vi "Init Module.vi"(8 "error in (no error) 4":errorcluster, 10 "UI COnfiguration  3":T2, 11 "DB Reference In":T4) -> (0 "error out":errorcluster)   [LabVIEW 2015, in "Copy of Untitled Library 1.lvlib"]
uses:
  Copy of Untitled Library 1.lvlib
  <vilib>/addons/database/Connection.llb/Conn ObjectReference.ctl
  <userlib>/origin_lib_main/userlogin_lib/Control/Queue and Caller MSG.ctl
  Controls/FGV Cluster Data.ctl
  Controls/Enum Constant.ctl
  <userlib>/origin_lib_main/ui_msg_lib/CTRL/Display MSG Types.ctl
  <vilib>/addons/database/Connection.llb/DB Tools Open Connec (String).vi
  <vilib>/addons/database/NI_Database_API.lvlib
  <userlib>/origin_lib_main/db_interface/DB Interface.lvlib
  <userlib>/origin_lib_main/ui_msg_lib/MSG Library.lvlib
panel:
  in  "Data In":T3
  in  "UI COnfiguration  2":T5
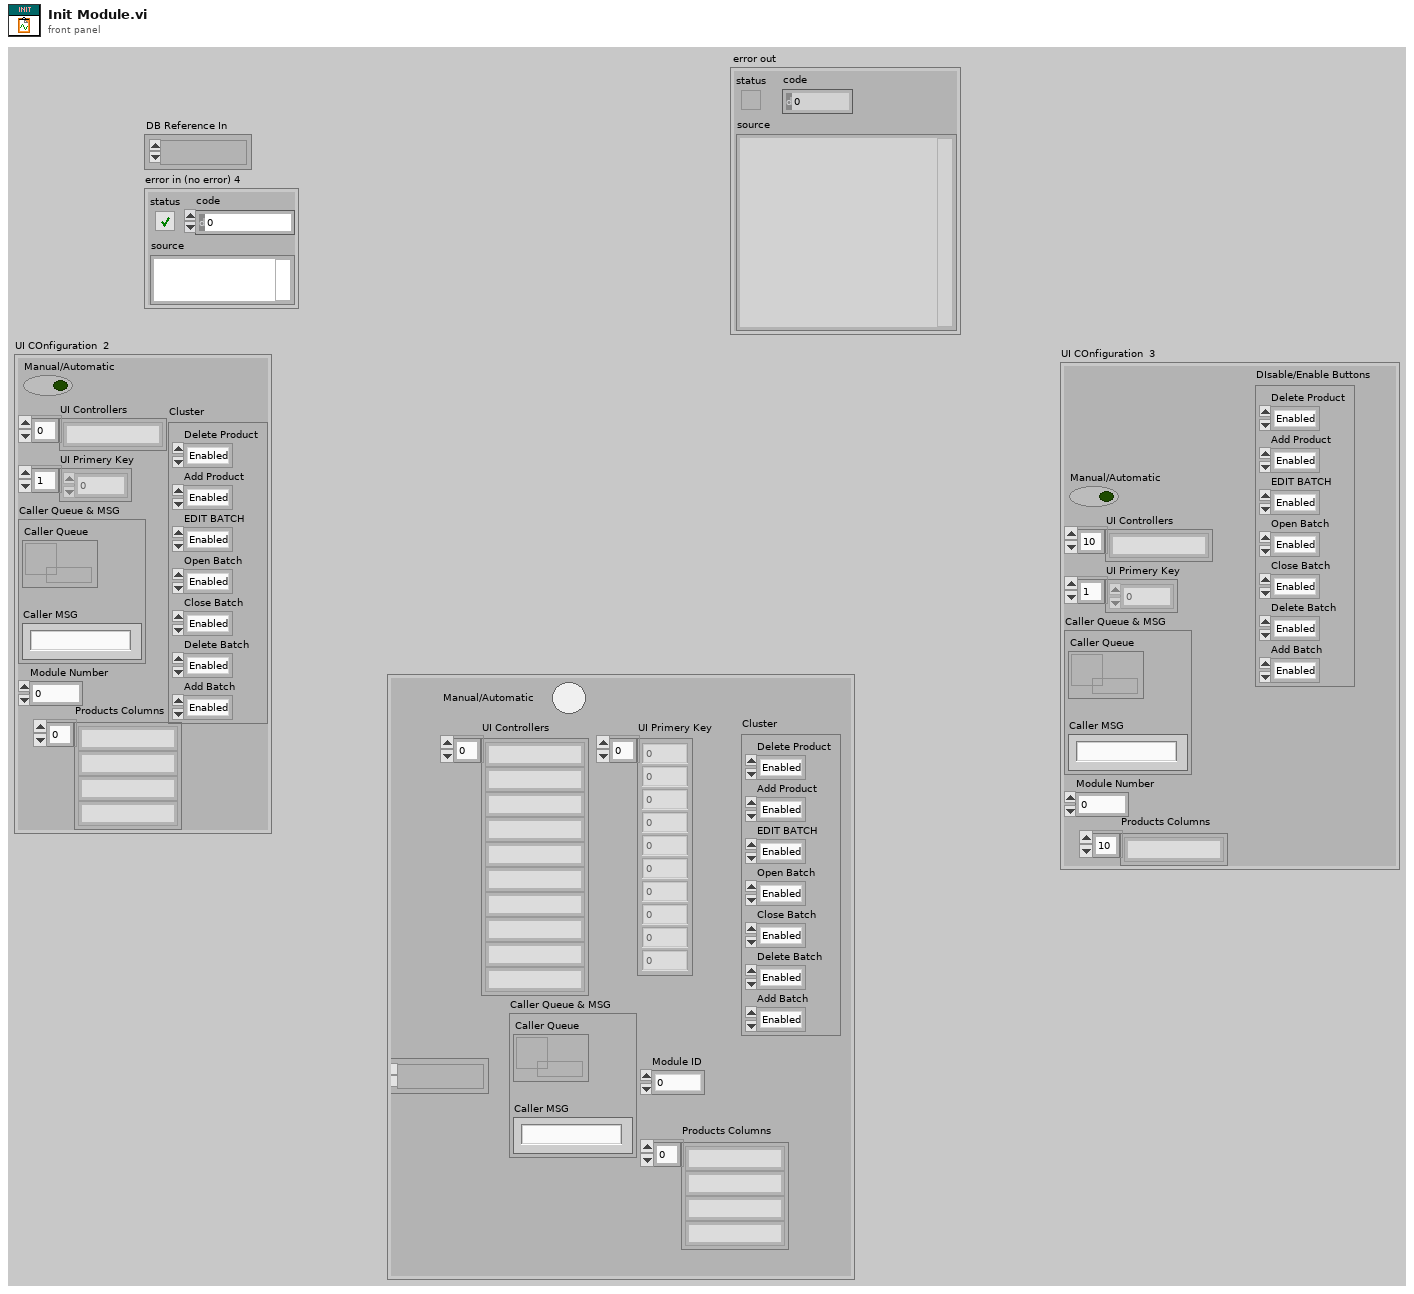
[diagram p1: front panel]
types:
  T1 = typedef "Queue and Caller MSG.ctl" = cluster{"Caller Queue":refnum<queue>, "Caller MSG":string}
  T2 = cluster{"Manual/Automatic":bool, "UI Controllers ":string[], "UI Primery Key ":dbl[], "Caller Queue & MSG":T1, "Module Number":dbl, "Products Columns":string[], "DIsable/Enable Buttons":cluster{"Delete Product":enum8{"Enabled", "Disabled", "Disabled and Grayed Out"}, "Add Product ":enum8{"Enabled", "Disabled", "Disabled and Grayed Out"}, "EDIT BATCH":enum8{"Enabled", "Disabled", "Disabled and Grayed Out"}, "Open Batch ":enum8{"Enabled", "Disabled", "Disabled and Grayed Out"}, "Close Batch":enum8{"Enabled", "Disabled", "Disabled and Grayed Out"}, "Delete Batch":enum8{"Enabled", "Disabled", "Disabled and Grayed Out"}, "Add Batch ":enum8{"Enabled", "Disabled", "Disabled and Grayed Out"}}}
  T3 = typedef "FGV Cluster Data.ctl" = cluster{"Manual/Automatic":bool, "UI Controllers ":string[], "UI Primery Key ":dbl[], "Caller Queue & MSG":T1, "Module ID":dbl, "DB Reference In":T4, "Products Columns":string[], "Cluster":cluster{"Delete Product":enum8{"Enabled", "Disabled", "Disabled and Grayed Out"}, "Add Product ":enum8{"Enabled", "Disabled", "Disabled and Grayed Out"}, "EDIT BATCH":enum8{"Enabled", "Disabled", "Disabled and Grayed Out"}, "Open Batch ":enum8{"Enabled", "Disabled", "Disabled and Grayed Out"}, "Close Batch":enum8{"Enabled", "Disabled", "Disabled and Grayed Out"}, "Delete Batch":enum8{"Enabled", "Disabled", "Disabled and Grayed Out"}, "Add Batch ":enum8{"Enabled", "Disabled", "Disabled and Grayed Out"}}}
  T4 = typedef "NI_Database_API.lvlib/Conn ObjectReference.ctl" = refnum<k1>
  T5 = cluster{"Manual/Automatic":bool, "UI Controllers ":string[], "UI Primery Key ":dbl[], "Caller Queue & MSG":T1, "Module Number":dbl, "Products Columns":string[], "Cluster":cluster{"Delete Product":enum8{"Enabled", "Disabled", "Disabled and Grayed Out"}, "Add Product ":enum8{"Enabled", "Disabled", "Disabled and Grayed Out"}, "EDIT BATCH":enum8{"Enabled", "Disabled", "Disabled and Grayed Out"}, "Open Batch ":enum8{"Enabled", "Disabled", "Disabled and Grayed Out"}, "Close Batch":enum8{"Enabled", "Disabled", "Disabled and Grayed Out"}, "Delete Batch":enum8{"Enabled", "Disabled", "Disabled and Grayed Out"}, "Add Batch ":enum8{"Enabled", "Disabled", "Disabled and Grayed Out"}}}
  T6 = enum32{"Bad", "Idle", "Run top level", "Running"}
  T7 = typedef "Enum Constant.ctl" = enum16{"Init", "Read", "Write"}
  T8 = typedef "MSG Library.lvlib/Display MSG Types.ctl" = enum16{"Display MSG 1", "Display MSG 2", "Display MSG Load", "End MSG Load ", "Display 2 STR MSG"}
  T9 = cluster{"Delete Product":enum8{"Enabled", "Disabled", "Disabled and Grayed Out"}, "Add Product ":enum8{"Enabled", "Disabled", "Disabled and Grayed Out"}, "EDIT BATCH":enum8{"Enabled", "Disabled", "Disabled and Grayed Out"}, "Open Batch ":enum8{"Enabled", "Disabled", "Disabled and Grayed Out"}, "Close Batch":enum8{"Enabled", "Disabled", "Disabled and Grayed Out"}, "Delete Batch":enum8{"Enabled", "Disabled", "Disabled and Grayed Out"}, "Add Batch ":enum8{"Enabled", "Disabled", "Disabled and Grayed Out"}}
  T10 = typedef "FGV Data.ctl" = T3[]
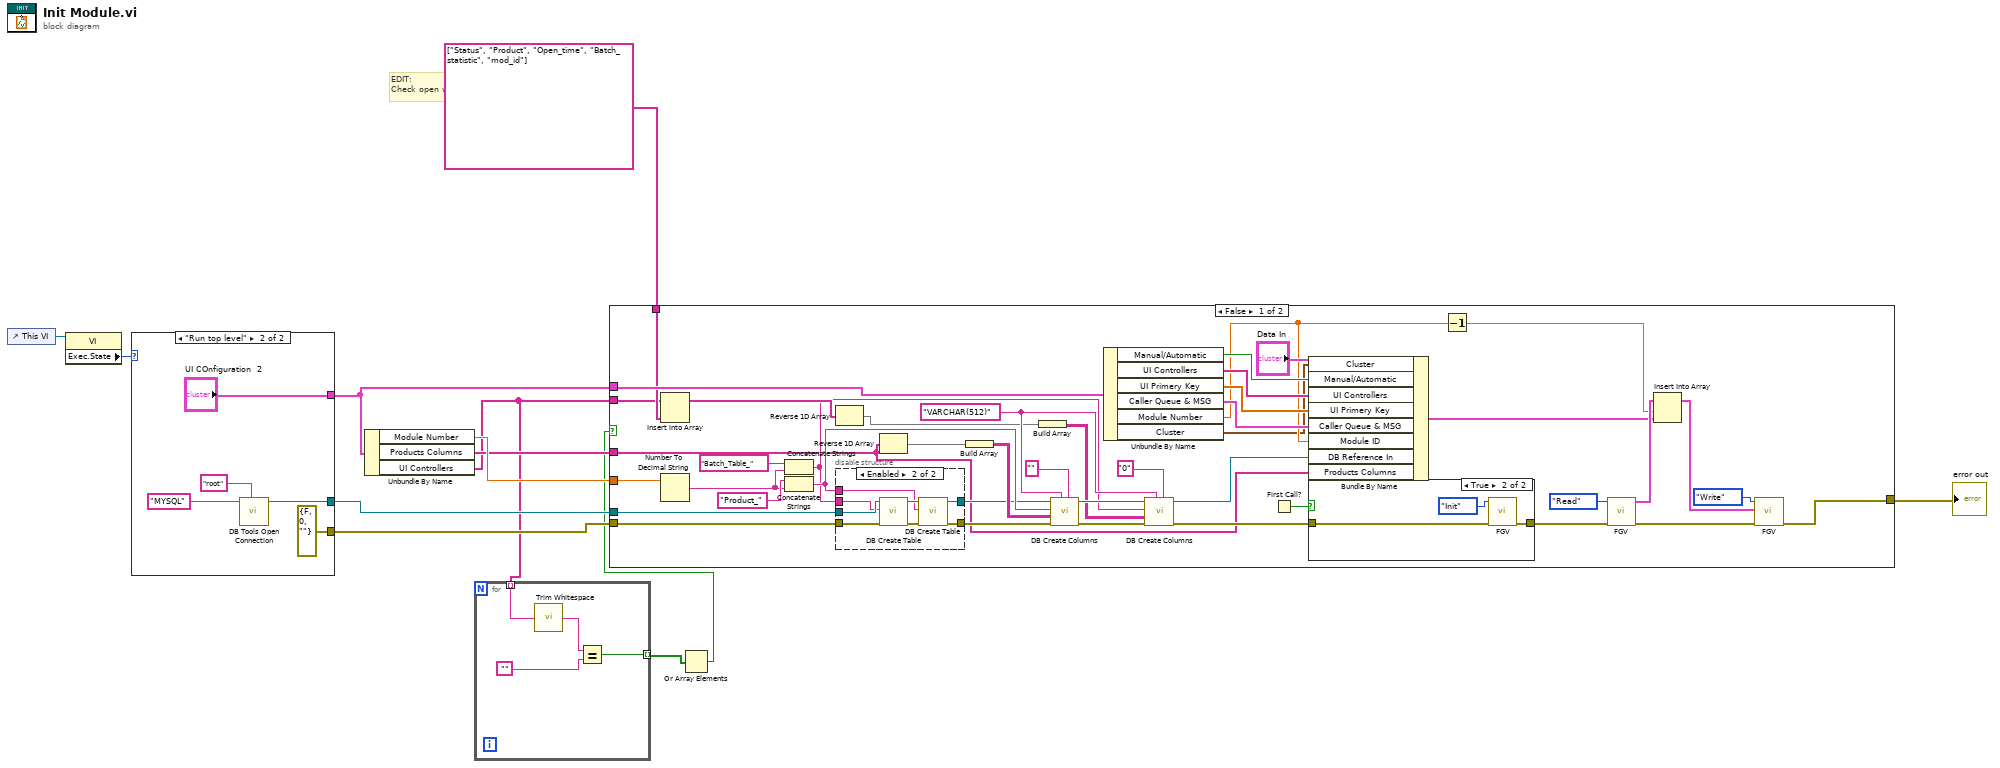
[diagram p0: block diagram]
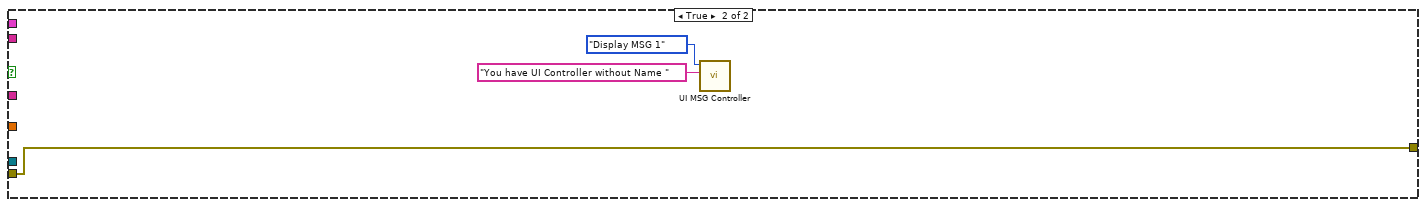
[diagram p4: hidden frame]
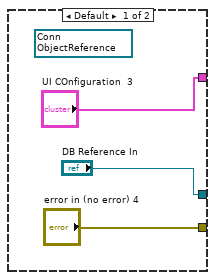
[diagram p5: hidden frame]
diagram:
  # "EDIT:\nCheck open with Mod_ID"
  n1 = control-ref of="This VI"() -> (w12:refnum<vi>)
  n2 = property class="VI"(reference=w12) -> ("Exec.State"=w11:T6)  [unwired: 1 in, 2 out]
  n3 = case shown="\"Run top level\"" w11 {
    tunnel: ["DB Reference In" w18] -> w7
    tunnel: ["error in (no error) 4" errorcluster {"status"=FALSE, "code"=0, "source"=""} ("error in (no error) 3")] -> w6
    tunnel: ["UI COnfiguration  3" "UI COnfiguration  2"] -> w10
    frame Default {
      (unwired) T4 refnum items=["Connection"] ("DB Reference In")
    }
    frame "Run top level" {
      n4 = call-poly <vilib>:"DB Tools Open Connection.vi"("userID"="root", "connection information"="MYSQL" ("userID")) -> ("connection reference"=w18:T4)  [unwired: 6 in, 1 out]
    }
  }
  n5 = Unbundle By Name(w10) -> ("Module Number"=w9:dbl, "Products Columns"=w5:string[], "UI Controllers"=w1:string[])
  n6 = for {
    tunnel: w1 -> [w24] mode=indexing
    tunnel: [w21] -> w4 mode=indexing
    n7 = call <vilib>:"Trim Whitespace.vi"("string"=w24) -> ("trimmed string"=w23:string)  [unwired: 1 in]
    n8 = Equal?(x=w23, y="") -> (x = y?=w21:bool)
  }
  n9 = Or Array Elements(Boolean array=w4) -> (logical OR=w3:bool)
  n10 = case shown="False" w3 {
    tunnel: w10 -> [w54 _]
    tunnel: w9 -> [w53 _]
    tunnel: string[] ["Status", "Product", "Open_time", "Batch_statistic", "mod_id"] ("element") -> [w40 _]
    tunnel: w1 -> [w39 _]
    tunnel: w7 -> [w32 _]
    tunnel: w6 -> [w31 w80]
    tunnel: w5 -> [w27 _]
    tunnel: [w26 w80] -> w2
    frame False {
      w46 = "VARCHAR(512)" ("Default Data Type")
      n11 = Insert Into Array(array=w39, new element=w40) -> (w38:string[])  [unwired: 1 in]
      n12 = Number To Decimal String(number=w53) -> (decimal integer string=w47:string)  [unwired: 1 in]
      n13 = Concatenate Strings("Batch_Table_" ("string"), w47) -> (w30:string)
      n14 = Concatenate Strings("Product_" ("string"), w47) -> (w33:string)
      n15 = Reverse 1D Array(array=w38) -> (reversed array=w37:string[])
      n16 = disable-structure shown="Enabled" {
        disable-tunnel: [_ w71] -> w29
        disable-tunnel: [_ w69] -> w28
        disable-tunnel: w32 -> [_ w75]
        disable-tunnel: w30 -> [_ w74]
        disable-tunnel: w33 -> [_ w72]
        disable-tunnel: w31 -> [_ w68]
        frame Disabled {
        }
        frame Enabled {
          n17 = call <userlib>:"DB Create Table.vi"("error in (no error)"=w68, "Table Name"=w74, "connection reference"=w75) -> ("error out"=w70:errorcluster, "connection reference 2"=w73:T4)  [unwired: 6 in, 1 out]
          n18 = call <userlib>:"DB Create Table.vi"("error in (no error)"=w70, "Table Name"=w72, "connection reference"=w73) -> ("error out"=w69:errorcluster, "connection reference 2"=w71:T4)  [unwired: 6 in, 1 out]
        }
      }
      n19 = Reverse 1D Array(array=w27) -> (reversed array=w52:string[])
      n20 = Build Array(w52) -> (w51:string[][])
      n21 = Build Array(w37) -> (w36:string[][])
      n22 = call <userlib>:"DB Create Columns.vi"("Default Default value"="", "Default Data Type"=w46, "error in (no error)"=w28, "Columns Config (Name;Datatype;Default;Unique?)"=w51, "Table to be added to"=w33, "connection reference in"=w29) -> ("error out"=w43:errorcluster, "connection reference out"=w49:T4)  [unwired: 2 in, 2 out]
      n23 = Unbundle By Name(w54) -> ("Manual/Automatic"=w64:bool, "UI Controllers"=w63:string[], "UI Primery Key"=w62:dbl[], "Caller Queue & MSG"=w61:T1, "Module Number"=w55:dbl, "Cluster"=w25:T9)
      n24 = call <userlib>:"DB Create Columns.vi"("Default Default value"="0", "Default Data Type"=w46, "error in (no error)"=w43, "Columns Config (Name;Datatype;Default;Unique?)"=w36, "Table to be added to"=w30, "connection reference in"=w49) -> ("error out"=w42:errorcluster, "connection reference out"=w41:T4)  [unwired: 2 in, 2 out]
      n25 = First Call?() -> (First Call?: T/F=w45:bool)
      n26 = Bundle By Name(cluster="Data In", "Cluster"=w25, "Manual/Automatic"=w64, "UI Controllers"=w63, "UI Primery Key"=w62, "Caller Queue & MSG"=w61, "Module ID"=w55, "DB Reference In"=w41, "Products Columns"=w27) -> (w60:T3)
      n27 = case shown="True" w45 {
        tunnel: [w76 w78] -> w44
        tunnel: w42 -> [w76 w77]
        frame False {
        }
        frame True {
          n28 = call "FGV.vi"("error out 2"=w77, "Enum"=Enum_Constant."Init") -> ("error out"=w78:errorcluster)  [unwired: 8 in, 1 out]
        }
      }
      n29 = Decrement(x=w55) -> (x-1=w56:dbl)
      n30 = call "FGV.vi"("error out 2"=w44, "Enum"=Enum_Constant."Read") -> ("error out"=w57:errorcluster, "Read Data"=w66:T10)  [unwired: 8 in]
      n31 = Insert Into Array(array=w66, index=w56, new element=w60) -> (w59:T10)
      n32 = call "FGV.vi"("error out 2"=w57, "Write Data"=w59, "Enum"=Enum_Constant."Write") -> ("error out"=w26:errorcluster)  [unwired: 7 in, 1 out]
    }
    frame True {
      n33 = call <userlib>:"UI MSG Controller.vi"("MSG"="You have UI Controller without Name ", "Display MSG Type"=Display_MSG_Types."Display MSG 1") -> ()  [unwired: 6 in, 4 out]
    }
  }
  "error out" <- w2
